vi "Globals to XML.vi"(8 "Array":path[](array[path])) -> ()   [LabVIEW 2020]
uses:
  <vilib>/Utility/xml.llb/Write to XML File(string).vi
  Globals/Dashboard_Cal_Globals.vi
  2021-MARS-Swerve/Globals/Intake_Globals.vi
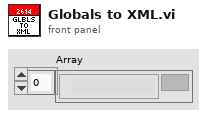
[diagram p1: front panel]
types:
  T1 = cluster{"Turret_Kd":dbl, "Turret_Ki":dbl, "Turret_Kp":dbl, "Turret_Lower_Limit":dbl, "Turret_Upper_Limit":dbl}
  T2 = cluster{"Magazine_Firing_Throttle":dbl, "Manual_Magazine_Power":dbl}
  T3 = cluster{"Flywheel_Acceptable_Error":dbl, "Flywheel_Speed_Multiplier":dbl}
  T4 = cluster{"FR_Kp":dbl, "FR_Ki":dbl, "FR_Kd":dbl, "FR_N-Diff":dbl, "FR_N-Int":dbl, "FR_Int Error Window":dbl, "FR_Max Output":dbl, "FR_Min Output":dbl, "FL_Kp":dbl, "FL_Ki":dbl, "FL_Kd":dbl, "FL_N-Diff":dbl, "FL_N-Int":dbl, "FL_Int Error Window":dbl, "FL_Max Output":dbl, "FL_Min Output":dbl, "BL_Kp":dbl, "BL_Ki":dbl, "BL_Kd":dbl, "BL_N-Diff":dbl, "BL_N-Int":dbl, "BL_Int Error Window":dbl, "BL_Max Output":dbl, "BL_Min Output":dbl, "BR_Kp":dbl, "BR_Ki":dbl, "BR_Kd":dbl, "BR_N-Diff":dbl, "BR_N-Int":dbl, "BR_Int Error Window":dbl, "BR_Max Output":dbl, "BR_Min Output":dbl}
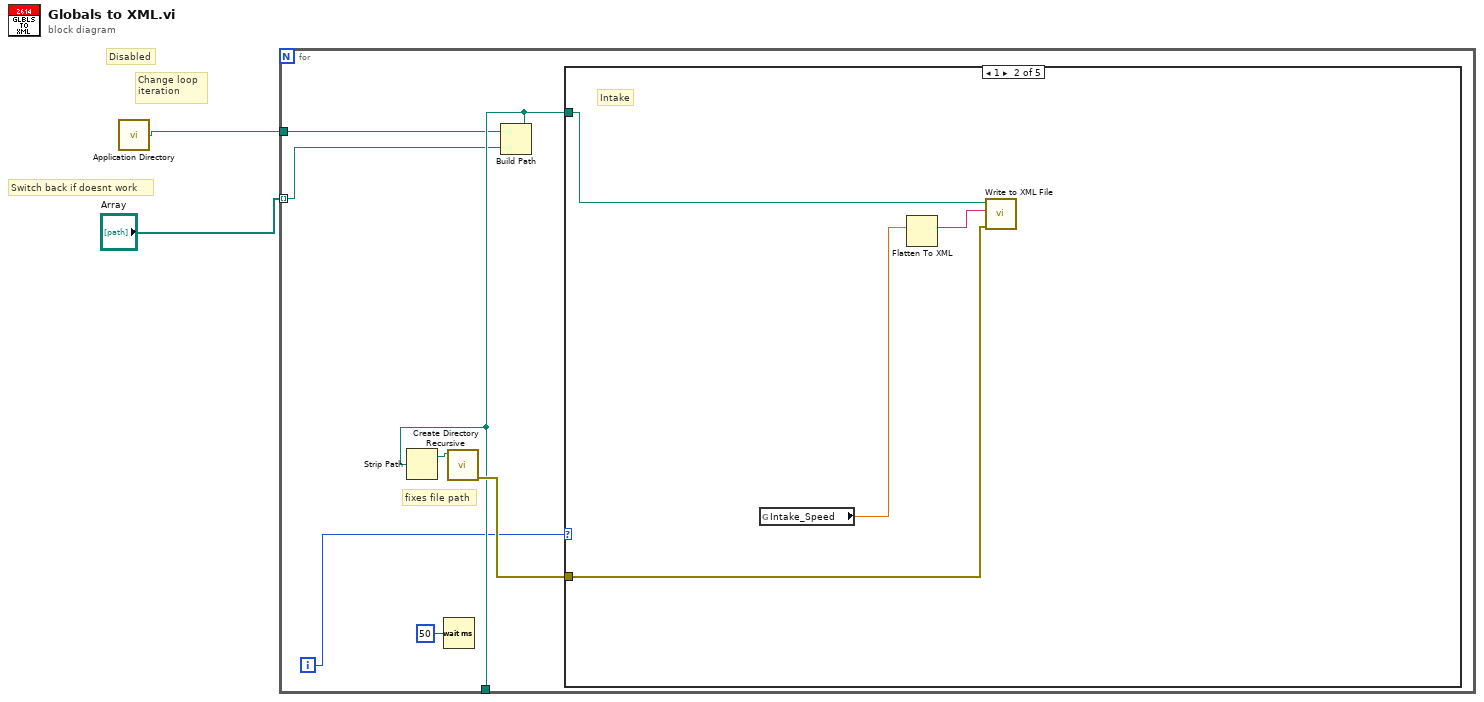
[diagram p0: block diagram]
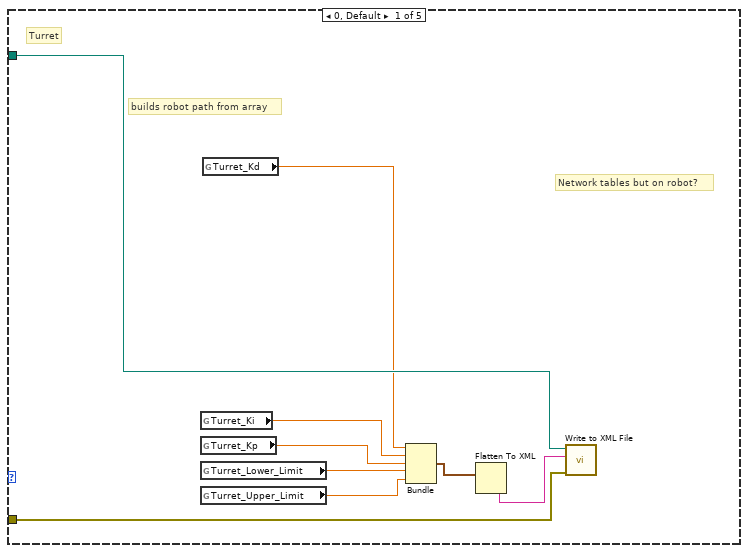
[diagram p2: hidden frame]
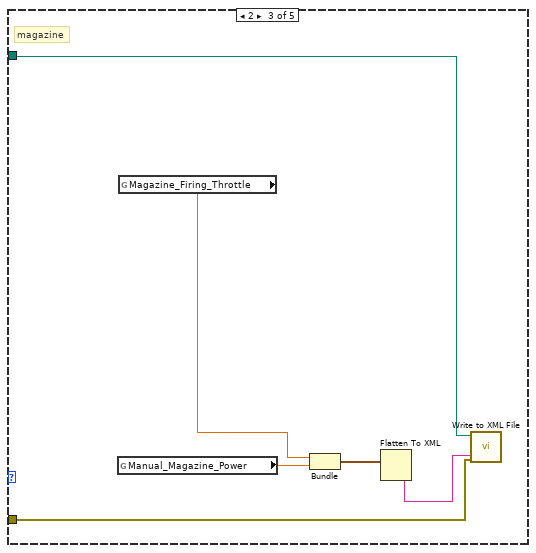
[diagram p3: hidden frame]
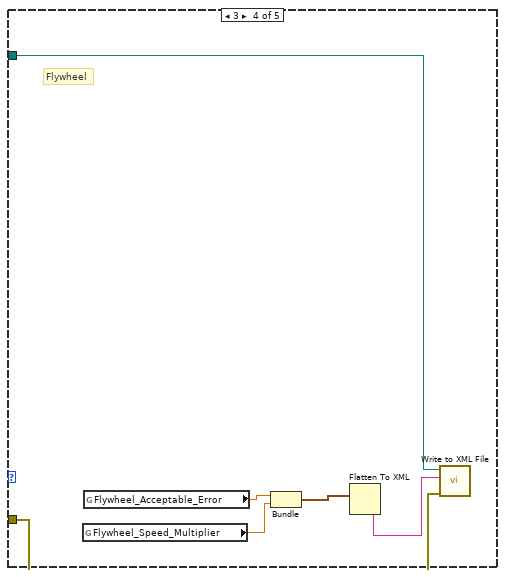
[diagram p4: hidden frame]
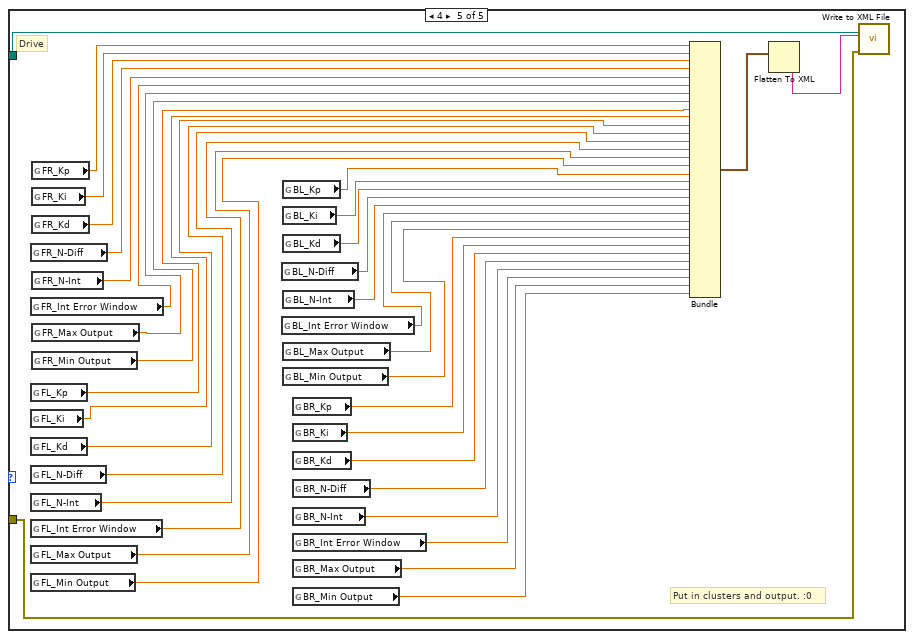
[diagram p5: hidden frame]
diagram:
  # "Switch back if doesnt work"
  # "Change loop\niteration"
  # "Disabled"
  n1 = call <vilib>:"Application Directory.vi"() -> ("Application Directory"=w2:path)
  n2 = for {
    tunnel: [w6] -> _
    tunnel: w2 -> [w5]
    tunnel: "Array" -> [w4] mode=indexing
    i -> [w3]
    # "fixes file path"
    n3 = Wait (ms)(milliseconds to wait=u32 50) -> ()  [unwired: 1 out]
    n4 = Build Path(base path=w5, name or relative path=w4) -> (appended path=w6:path)
    n5 = Strip Path(path=w6) -> (stripped path=w8:path)  [unwired: 1 out]
    n6 = call <vilib>:"Create Directory Recursive.vi"("directory"=w8) -> ("error out"=w7:errorcluster)  [unwired: 4 in, 2 out]
    n7 = case shown="1" w3 {
      tunnel: w6 -> [w17 w21 w26 w34 w69]
      tunnel: w7 -> [w16 w20 w23 w30 w62]
      frame 0, Default {
        # "Network tables but on robot?"
        # "builds robot path from array"
        # "Turret"
        n8 = global read "Dashboard_Cal_Globals.vi" "Turret_Ki"() -> (w14:dbl)
        n9 = global read "Dashboard_Cal_Globals.vi" "Turret_Kp"() -> (w13:dbl)
        n10 = global read "Dashboard_Cal_Globals.vi" "Turret_Lower_Limit"() -> (w12:dbl)
        n11 = global read "Dashboard_Cal_Globals.vi" "Turret_Upper_Limit"() -> (w11:dbl)
        n12 = global read "Dashboard_Cal_Globals.vi" "Turret_Kd"() -> (w15:dbl)
        n13 = Bundle("Turret_Kd"=w15, "Turret_Ki"=w14, "Turret_Kp"=w13, "Turret_Lower_Limit"=w12, "Turret_Upper_Limit"=w11) -> (w18:T1)  [unwired: 1 in]
        n14 = Flatten To XML(anything=w18) -> (xml string=w10:string)
        n15 = call-poly <vilib>:"Write to XML File.vi"("error in (no error)"=w16, "XML Input"=w10, "XML File Path"=w17) -> ()  [unwired: 6 in, 3 out]
      }
      frame 1 {
        # "Intake"
        n16 = global read "Intake_Globals.vi" "Intake_Speed"() -> (w22:dbl)
        n17 = Flatten To XML(anything=w22) -> (xml string=w19:string)
        n18 = call-poly <vilib>:"Write to XML File.vi"("error in (no error)"=w20, "XML Input"=w19, "XML File Path"=w21) -> ()  [unwired: 6 in, 3 out]
      }
      frame 2 {
        # "magazine"
        n19 = global read "Dashboard_Cal_Globals.vi" "Manual_Magazine_Power"() -> (w24:dbl)
        n20 = global read "Dashboard_Cal_Globals.vi" "Magazine_Firing_Throttle"() -> (w25:dbl)
        n21 = Bundle("Magazine_Firing_Throttle"=w25, "Manual_Magazine_Power"=w24) -> (w27:T2)  [unwired: 1 in]
        n22 = Flatten To XML(anything=w27) -> (xml string=w28:string)
        n23 = call-poly <vilib>:"Write to XML File.vi"("error in (no error)"=w23, "XML Input"=w28, "XML File Path"=w26) -> ()  [unwired: 6 in, 3 out]
      }
      frame 3 {
        # "Flywheel"
        n24 = global read "Dashboard_Cal_Globals.vi" "Flywheel_Speed_Multiplier"() -> (w31:dbl)
        n25 = global read "Dashboard_Cal_Globals.vi" "Flywheel_Acceptable_Error"() -> (w32:dbl)
        n26 = Bundle("Flywheel_Acceptable_Error"=w32, "Flywheel_Speed_Multiplier"=w31) -> (w33:T3)  [unwired: 1 in]
        n27 = Flatten To XML(anything=w33) -> (xml string=w29:string)
        n28 = call-poly <vilib>:"Write to XML File.vi"("error in (no error)"=w30, "XML Input"=w29, "XML File Path"=w34) -> ()  [unwired: 6 in, 3 out]
      }
      frame 4 {
        # "Put in clusters and output. :0"
        # "Drive"
        n29 = global read "Dashboard_Cal_Globals.vi" "FR_N-Diff"() -> (w43:dbl)
        n30 = global read "Dashboard_Cal_Globals.vi" "FR_Int Error Window"() -> (w41:dbl)
        n31 = global read "Dashboard_Cal_Globals.vi" "FL_Kp"() -> (w38:dbl)
        n32 = global read "Dashboard_Cal_Globals.vi" "FL_Ki"() -> (w37:dbl)
        n33 = global read "Dashboard_Cal_Globals.vi" "FL_Kd"() -> (w36:dbl)
        n34 = global read "Dashboard_Cal_Globals.vi" "FL_N-Diff"() -> (w68:dbl)
        n35 = global read "Dashboard_Cal_Globals.vi" "FL_N-Int"() -> (w67:dbl)
        n36 = global read "Dashboard_Cal_Globals.vi" "FL_Int Error Window"() -> (w66:dbl)
        n37 = global read "Dashboard_Cal_Globals.vi" "FL_Max Output"() -> (w65:dbl)
        n38 = global read "Dashboard_Cal_Globals.vi" "FL_Min Output"() -> (w64:dbl)
        n39 = global read "Dashboard_Cal_Globals.vi" "FR_Kp"() -> (w46:dbl)
        n40 = global read "Dashboard_Cal_Globals.vi" "FR_Ki"() -> (w45:dbl)
        n41 = global read "Dashboard_Cal_Globals.vi" "FR_Kd"() -> (w44:dbl)
        n42 = global read "Dashboard_Cal_Globals.vi" "FR_N-Int"() -> (w42:dbl)
        n43 = global read "Dashboard_Cal_Globals.vi" "FR_Max Output"() -> (w40:dbl)
        n44 = global read "Dashboard_Cal_Globals.vi" "FR_Min Output"() -> (w39:dbl)
        n45 = global read "Dashboard_Cal_Globals.vi" "BL_N-Diff"() -> (w59:dbl)
        n46 = global read "Dashboard_Cal_Globals.vi" "BL_Int Error Window"() -> (w57:dbl)
        n47 = global read "Dashboard_Cal_Globals.vi" "BL_Kp"() -> (w63:dbl)
        n48 = global read "Dashboard_Cal_Globals.vi" "BL_Ki"() -> (w61:dbl)
        n49 = global read "Dashboard_Cal_Globals.vi" "BL_Kd"() -> (w60:dbl)
        n50 = global read "Dashboard_Cal_Globals.vi" "BL_N-Int"() -> (w58:dbl)
        n51 = global read "Dashboard_Cal_Globals.vi" "BL_Max Output"() -> (w56:dbl)
        n52 = global read "Dashboard_Cal_Globals.vi" "BL_Min Output"() -> (w55:dbl)
        n53 = global read "Dashboard_Cal_Globals.vi" "BR_Kp"() -> (w54:dbl)
        n54 = global read "Dashboard_Cal_Globals.vi" "BR_Ki"() -> (w53:dbl)
        n55 = global read "Dashboard_Cal_Globals.vi" "BR_Kd"() -> (w52:dbl)
        n56 = global read "Dashboard_Cal_Globals.vi" "BR_N-Diff"() -> (w51:dbl)
        n57 = global read "Dashboard_Cal_Globals.vi" "BR_N-Int"() -> (w50:dbl)
        n58 = global read "Dashboard_Cal_Globals.vi" "BR_Int Error Window"() -> (w49:dbl)
        n59 = global read "Dashboard_Cal_Globals.vi" "BR_Max Output"() -> (w48:dbl)
        n60 = global read "Dashboard_Cal_Globals.vi" "BR_Min Output"() -> (w47:dbl)
        n61 = Bundle("FR_Kp"=w46, "FR_Ki"=w45, "FR_Kd"=w44, "FR_N-Diff"=w43, "FR_N-Int"=w42, "FR_Int Error Window"=w41, "FR_Max Output"=w40, "FR_Min Output"=w39, "FL_Kp"=w38, "FL_Ki"=w37, "FL_Kd"=w36, "FL_N-Diff"=w68, "FL_N-Int"=w67, "FL_Int Error Window"=w66, "FL_Max Output"=w65, "FL_Min Output"=w64, "BL_Kp"=w63, "BL_Ki"=w61, "BL_Kd"=w60, "BL_N-Diff"=w59, "BL_N-Int"=w58, "BL_Int Error Window"=w57, "BL_Max Output"=w56, "BL_Min Output"=w55, "BR_Kp"=w54, "BR_Ki"=w53, "BR_Kd"=w52, "BR_N-Diff"=w51, "BR_N-Int"=w50, "BR_Int Error Window"=w49, "BR_Max Output"=w48, "BR_Min Output"=w47) -> (w70:T4)  [unwired: 1 in]
        n62 = Flatten To XML(anything=w70) -> (xml string=w35:string)
        n63 = call-poly <vilib>:"Write to XML File.vi"("error in (no error)"=w62, "XML Input"=w35, "XML File Path"=w69) -> ()  [unwired: 6 in, 3 out]
      }
    }
  }
